vi "Get Peaks Time.vi"(6 "dt":dbl, 9 "sp time":timestamp, 10 "Best fit results":dbl[][](array[numeric]) format="%#_4p", 11 "Frequency":dbl[](array[numeric])) -> (3 "Peaks absolute time":dbl[](array[numeric]))   [LabVIEW 2016]
panel:
  # "F0         dF     Ampl   Phase   Xbgrd   Ybgrd"
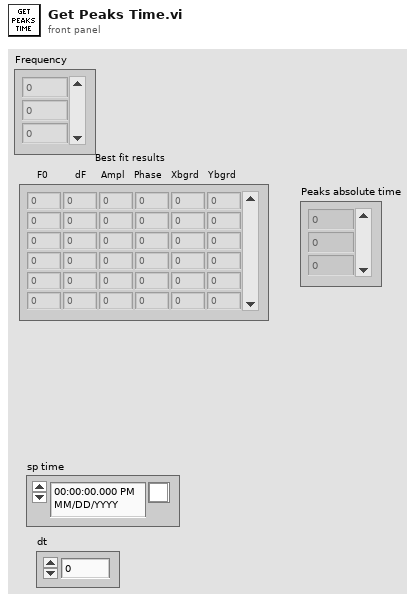
[diagram p1: front panel]
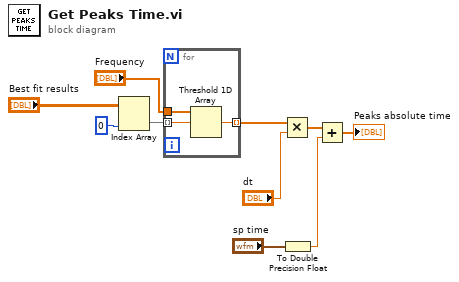
[diagram p0: block diagram]
diagram:
  n1 = Index Array(array="Best fit results", index (col)=0 ("disabled index (col)")) -> (element=w8:dbl[])  [unwired: 1 in]
  n2 = for {
    tunnel: w8 -> [w13] mode=indexing
    tunnel: "Frequency" -> [w12]
    tunnel: [w11] -> w6 mode=indexing
    n3 = Threshold 1D Array(2:w13, 3:w12) -> (0:w11:dbl)  [unwired: 1 in]
  }
  n4 = Multiply(x=w6, y="dt") -> (x*y=w2:dbl[])
  n5 = To Double Precision Float(number="sp time") -> (double precision float=w3:dbl)
  n6 = Add(x=w2, y=w3) -> (x+y=→"Peaks absolute time":dbl[])
